vi "Init.vi"(8 "error in (no error)":errorcluster, 10 "Node Reg":refnum<k20>, 11 "Node in":refnum<class "Node.lvclass">) -> (0 "error out":errorcluster, 3 "Node out":refnum<class "Node.lvclass">)   [LabVIEW 2025, in "Node.lvclass"]
uses:
  Node.lvclass
  Node.lvclass/Node.ctl
  Terminal.ctl
  <vilib>/xml/NI_XML.lvlib
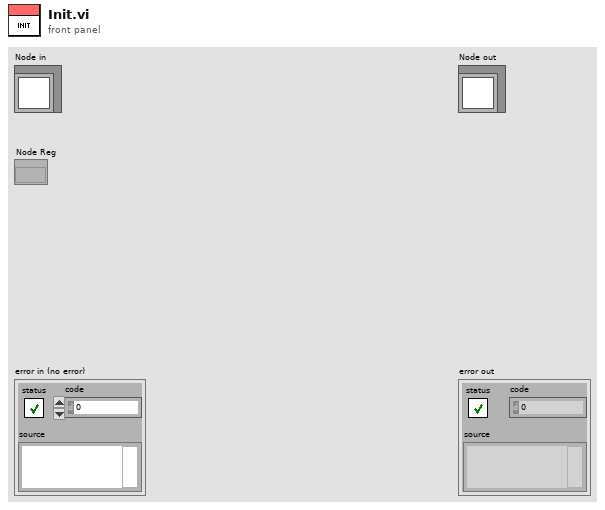
[diagram p1: front panel]
types:
  T1 = typedef "Terminal.ctl" = cluster{"id":string, "name":string, "terminal":refnum<vi>}
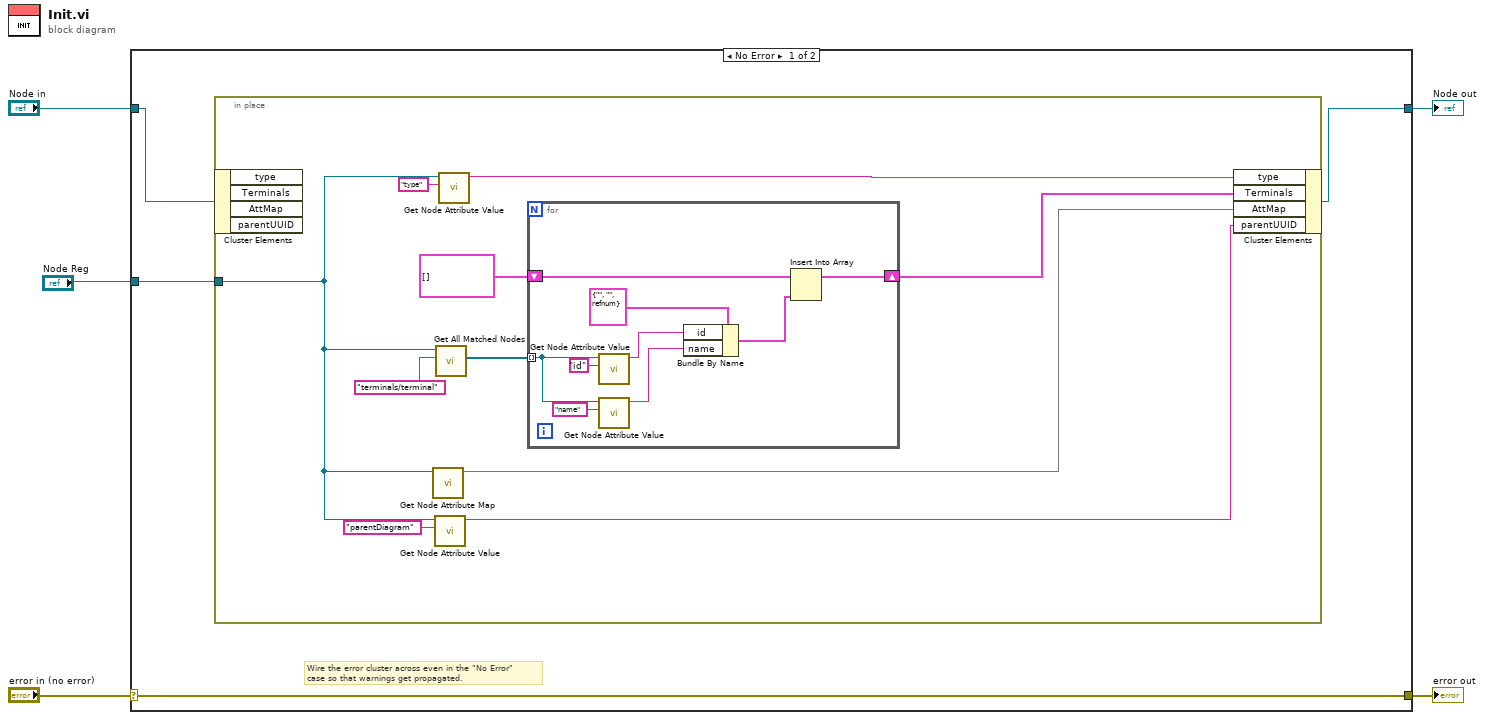
[diagram p0: block diagram]
diagram:
  n1 = case shown="No Error" "error in (no error)" {
    selector: "error in (no error)" -> [w9 w30]
    tunnel: [w9 w30] -> w4
    tunnel: [w6 w29] -> w2
    tunnel: "Node in" -> [w8 w29]
    tunnel: "Node Reg" -> [w7 _]
    frame No Error {
      # "Wire the error cluster across even in the \"No Error\"\ncase so that warnings get propagated."
      n2 = in-place {
        in-place-border: w7 -> [w12]
        n3 = in-place-cluster #1(w8) -> ()  [unwired: 4 out]
        n4 = call "Get Node Attribute Map.vi"("Refnum in"=w12) -> ("Map"=w18:map{string, string})  [unwired: 10 in]
        n5 = call "Get Node Attribute Value.vi"("Attribute Name"="parentDiagram", "Refnum in"=w12) -> ("Value"=w10:string)  [unwired: 9 in]
        n6 = call <vilib>:"Get All Matched Nodes.vi"("XPath expression"="terminals/terminal", "node in"=w12) -> ("node result array"=w15:refnum<k20>[])  [unwired: 7 in, 2 out]
        n7 = call "Get Node Attribute Value.vi"("Attribute Name"="type", "Refnum in"=w12) -> ("Value"=w17:string)  [unwired: 9 in]
        n8 = for {
          tunnel: w15 -> [w26] mode=indexing
          shift-right: [w27] -> w13
          shift-left: T1[] [] ("Terminals") -> [w28]
          n9 = call "Get Node Attribute Value.vi"("Attribute Name"="id", "Refnum in"=w26) -> ("Value"=w21:string)  [unwired: 9 in]
          n10 = call "Get Node Attribute Value.vi"("Attribute Name"="name", "Refnum in"=w26) -> ("Value"=w20:string)  [unwired: 9 in]
          n11 = Bundle By Name(cluster=T1 {"id"="", "name"="", "terminal"=refnum} ("Terminal"), "id"=w21, "name"=w20) -> (w22:T1)
          n12 = Insert Into Array(array=w28, new element=w22) -> (w27:T1[])  [unwired: 1 in]
        }
        n13 = in-place-cluster #1("type"=w17, "Terminals"=w13, "AttMap"=w18, "parentUUID"=w10) -> (w6:refnum<class "Node.lvclass">)
      }
    }
    frame Error {
    }
  }
  "error out" <- w4
  "Node out" <- w2
